vi "PopUp_Edit Resource.vi"(8 "error in (no error)":errorcluster, 11 "Resource in":T1) -> (0 "error out":errorcluster, 2 "OK Pressed?":bool, 3 "Resource out":T1)   [LabVIEW 2013, in "SET Project Editor.lvlib"]
uses:
  SET Project Editor.lvlib
  SET Project Data/Types/ProjFile_Resource Entry.ctl
  DialogEnum.ctl
  Lib/Unicode/SET_Unicode Tools.lvlib
  SET Project Data/SET Project Data.lvlib
panel:
  in  "Default Text":string
  in  "Tag":string
  in  "Cancel":bool
  in  "OK":bool
  # "Shared Resource"
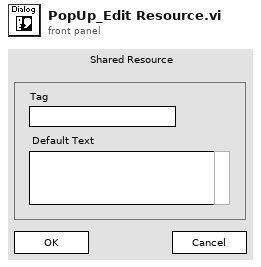
[diagram p1: front panel]
types:
  T1 = typedef "SET Project Data.lvlib/ProjFile_Resource Entry.ctl" = cluster{"RID":string, "Tag":string, "Strings [] (UTF-16)":string[], "Shared?":bool}
  T2 = typedef "SET Project Editor.lvlib/DialogEnum.ctl" = enum16{"Idle", "Init", "Shutdown"}
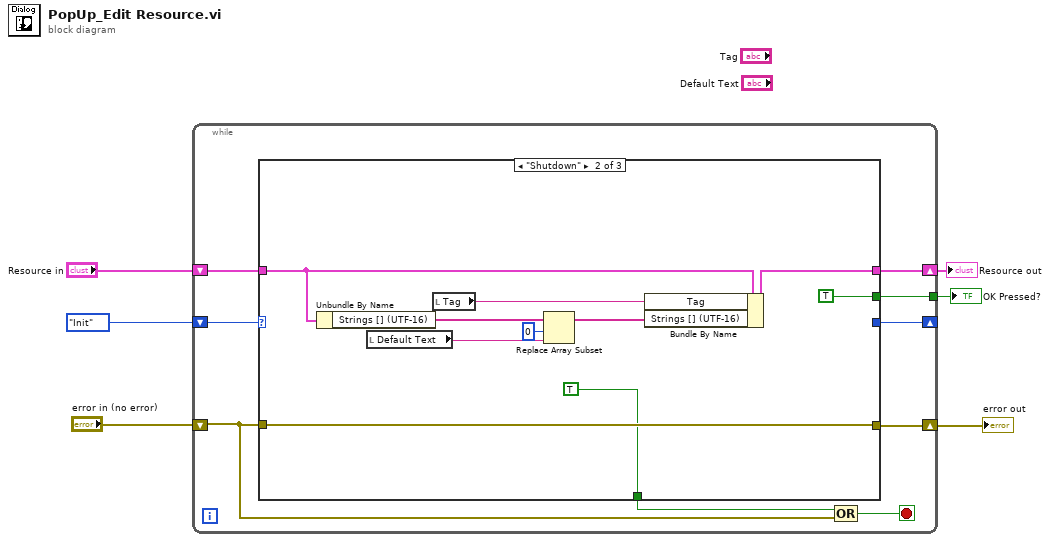
[diagram p0: block diagram]
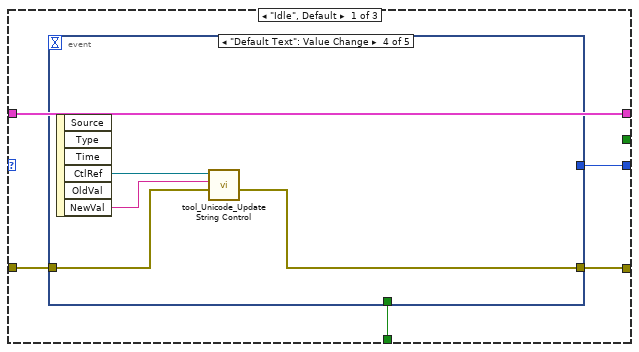
[diagram p2: hidden frame]
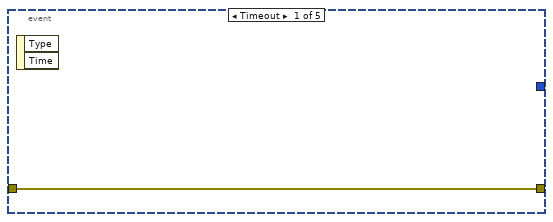
[diagram p3: hidden frame]
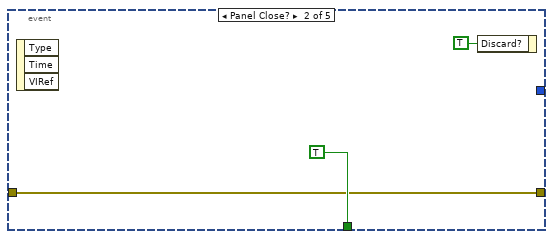
[diagram p4: hidden frame]
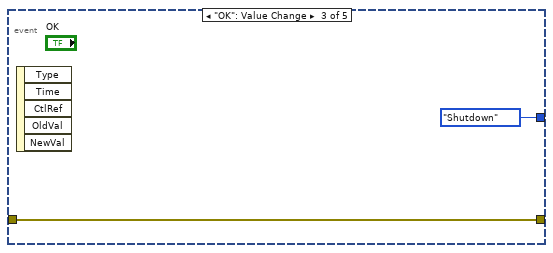
[diagram p5: hidden frame]
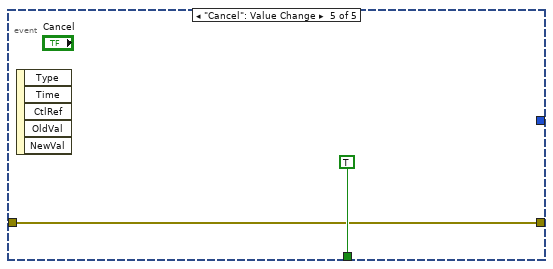
[diagram p6: hidden frame]
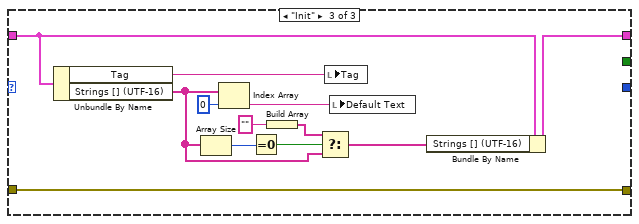
[diagram p7: hidden frame]
diagram:
  n1 = while {
    shift-right: [w14] -> w4
    shift-left: "error in (no error)" -> [w11]
    shift-right: [w13] -> _
    shift-left: DialogEnum."Init" -> [w15]
    shift-right: [w8] -> w2
    shift-left: "Resource in" -> [w9]
    tunnel: [w7] -> w1
    stop <- w10 stop-if-true
    n2 = case shown="\"Shutdown\"" w15 {
      tunnel: [w20 w42 w54] -> w14
      tunnel: w11 -> [w19 w42 w54]
      tunnel: [w18 TRUE _] -> w12
      tunnel: [w17 _ _] -> w13
      tunnel: w9 -> [w16 w40 w45]
      tunnel: [w16 w38 w44] -> w8
      tunnel: [_ TRUE _] -> w7
      frame "Idle", Default {
        n3 = event shown="[3] \"Default Text\": Value Change" {
          selector: _ -> [_ _ _ _ _]
          dyn-events: _ -> [_ _ _ _ _]
          timeout: _ -> [_ _ _ _ _]
          tunnel: [w21 w22 w25 w27 w31] -> w20
          tunnel: w19 -> [w21 w22 w25 w28 w31]
          tunnel: [_ TRUE _ _ TRUE] -> w18
          tunnel: [_ _ DialogEnum."Shutdown" _ _] -> w17
          event Timeout {
            n4 = event-data() -> ()  [unwired: 1 in, 2 out]
          }
          event Panel Close? {
            n5 = event-data() -> ()  [unwired: 1 in, 3 out]
            n6 = event-data("Discard?"=TRUE) -> ()  [unwired: 1 in, 1 out]
          }
          event "OK": Value Change {
            n7 = event-data() -> ()  [unwired: 1 in, 5 out]
          }
          event "Default Text": Value Change {
            n8 = event-data() -> ("CtlRef"=w30:refnum<vi>, "NewVal"=w29:string)  [unwired: 1 in, 4 out]
            n9 = call "tool_Unicode_Update String Control.vi"("error in (no error)"=w28, "String (UTF-16)"=w29, "*StrControl in"=w30) -> ("error out"=w27:errorcluster)  [unwired: 7 in, 1 out]
          }
          event "Cancel": Value Change {
            n10 = event-data() -> ()  [unwired: 1 in, 5 out]
          }
        }
      }
      frame "Shutdown" {
        n11 = Unbundle By Name(w40) -> ("Strings [] (UTF-16)"=w35:string[])
        n12 = local read "Default Text"() -> (w36:string)
        n13 = local read "Tag"() -> (w39:string)
        n14 = Replace Array Subset(array=w35, new element=w36, index=0) -> (w34:string[])
        n15 = Bundle By Name(cluster=w40, "Tag"=w39, "Strings [] (UTF-16)"=w34) -> (w38:T1)
      }
      frame "Init" {
        n16 = Unbundle By Name(w45) -> ("Tag"=w53:string, "Strings [] (UTF-16)"=w46:string[])
        n17 = Array Size(array=w46) -> (size(s)=w50:i32)
        n18 = Index Array(array=w46, index=0) -> (element=w52:string)
        n19 = Equal To 0?(x=w50) -> (x = 0?=w48:bool)
        n20 = Build Array("") -> (w47:string[])
        n21 = Select(t=w47, s=w48, f=w46) -> (s? t:f=w43:string[])
        n22 = local write "Tag"(w53) -> ()
        n23 = local write "Default Text"(w52) -> ()
        n24 = Bundle By Name(cluster=w45, "Strings [] (UTF-16)"=w43) -> (w44:T1)
      }
    }
    n25 = Compound Arithmetic op=OR(w12, w11) -> (w10:bool)
  }
  "error out" <- w4
  "Resource out" <- w2
  "OK Pressed?" <- w1
